vi "Vector-valued Function.vi"(1 "(x_1,...,x_n)":refnum<class "Dual.lvclass">[](array[class])) -> (0 "(f_1,...,f_n)":refnum<class "Dual.lvclass">[](array[class]))   [LabVIEW 2020, in "Tests.lvlib"]
uses:
  Tests.lvlib
  b6a85ad5-626d-4058-b824-40ffbd868fc6.vi
  1af88e31-763d-4e75-a921-d55d73349e85.vi
  72b3d7e6-e7b9-468f-a967-6ec54929e0e8.vi
  0232c1de-646f-48a7-bb7d-f7f53221b374.vi
  6f97315e-7bac-45fb-98c9-d02ae5ecc296.vi
  5b5ab934-7854-4bd5-a8aa-0cbb074ab388.vi
  classes/Dual/Dual.lvclass
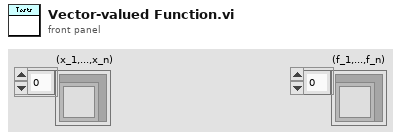
[diagram p1: front panel]
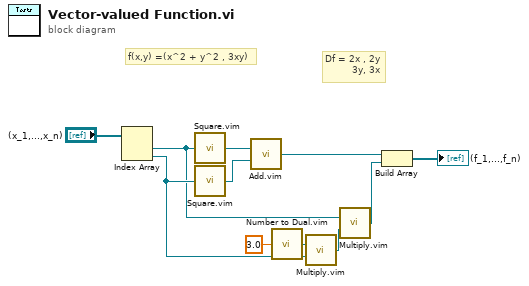
[diagram p0: block diagram]
diagram:
  # "Df = 2x , 2y\n         3y, 3x"
  # "f(x,y) =(x^2 + y^2 , 3xy)"
  n1 = Index Array(array="(x_1,...,x_n)") -> (element #1=w6:refnum<class "Dual.lvclass">, element #2=w7:refnum<class "Dual.lvclass">)  [unwired: 2 in]
  n2 = call "Square.vim"("x"=w6) -> ("x^2"=w11:refnum<class "Dual.lvclass">)
  n3 = call "Square.vim"("x"=w7) -> ("x^2"=w10:refnum<class "Dual.lvclass">)
  n4 = call "Add.vim"("x"=w11, "y"=w10) -> ("x + y"=w3:refnum<class "Dual.lvclass">)  [unwired: 13 in]
  n5 = call "Number to Dual.vim"("Number"=3.0 ("Double")) -> ("Dual"=w1:refnum<class "Dual.lvclass">)
  n6 = call "Multiply.vim"("x"=w1, "y"=w7) -> ("x * y"=w5:refnum<class "Dual.lvclass">)  [unwired: 13 in]
  n7 = call "Multiply.vim"("x"=w6, "y"=w5) -> ("x * y"=w4:refnum<class "Dual.lvclass">)  [unwired: 13 in]
  n8 = Build Array(w3, w4) -> (→"(f_1,...,f_n)":refnum<class "Dual.lvclass">[])
